vi "widget.vi"() -> ()   [LabVIEW 2018]
uses:
  <vilib>/Instr/_visa.llb/VISA Configure Serial Port (Instr).vi
  PCI8552B_32.dll
panel:
  out "待读取数据长度":i32
  out "步进电机步进次数":dbl
  out "频率步进次数":dbl
  in  "步进电机确定":bool
  in  "频率确定":bool
  in  "开关确定":bool
  in  "开始":bool
  in  "停止":bool
  in  "扫描模式":u16(ring)=2 items=["多频多角度模式", "校正模式", "单点模式", "单列模式", "单频多角度模式"]
  out "ch1":dbl[](graph)
  out "ch0":dbl[](graph)
  out "采集卡状态":bool
  out "开关控制器状态":bool
  out "步进电机控制器状态":bool
  in  "物体距离":dbl=150.0
  in  "频率间隔":dbl=0.1
  in  "步进间隔":dbl=5.0
  in  "移动坐标":dbl
  in  "改变频率":dbl
  in  "切换开关":dbl
  out "当前位置":dbl format="%#_4f"
  out "当前开关":dbl=1.0
  out "当前频率":dbl=24.0
  in  "开关控制器":refnum<visa-resource-name>
  in  "步进电机控制器":refnum<visa-resource-name>
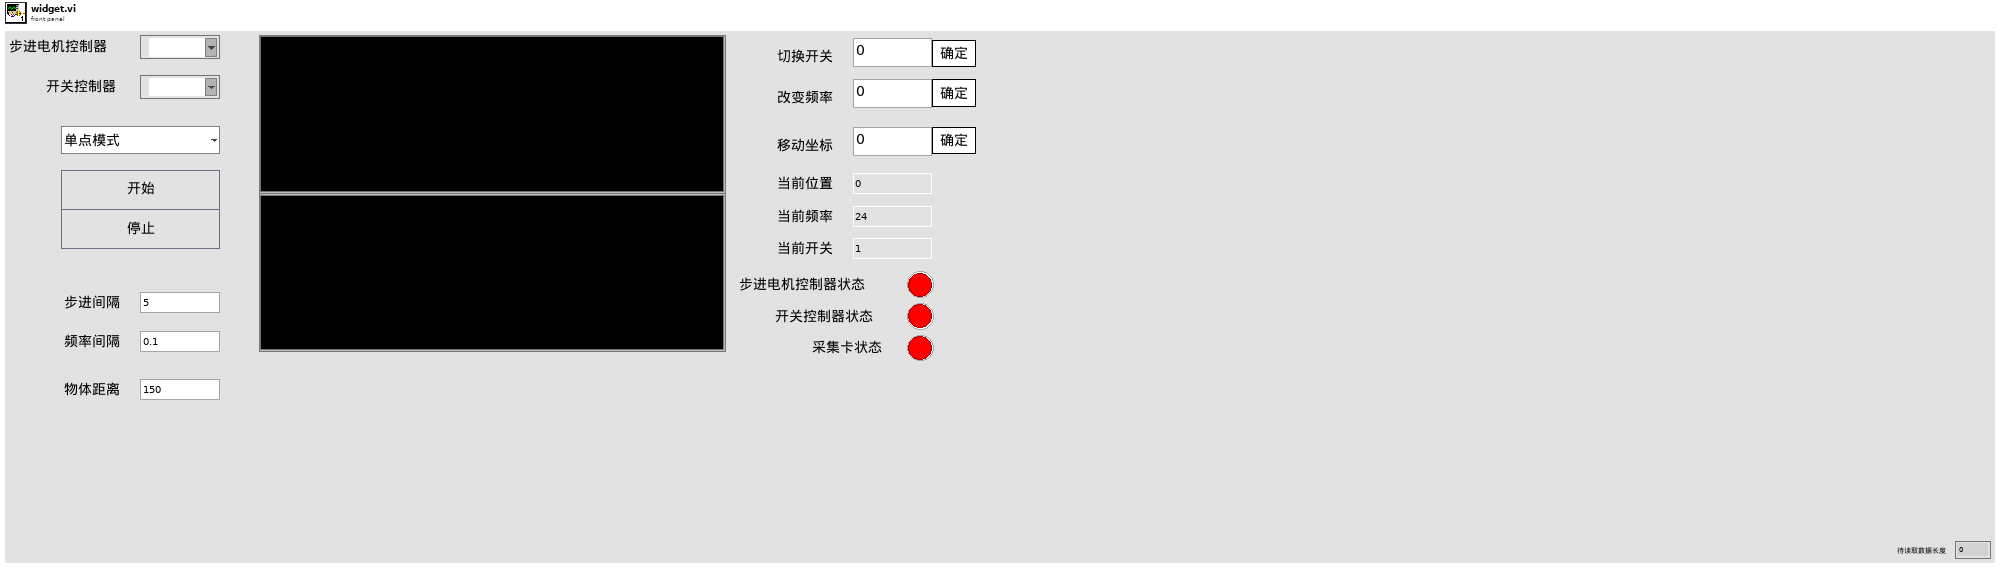
[diagram p1: front panel]
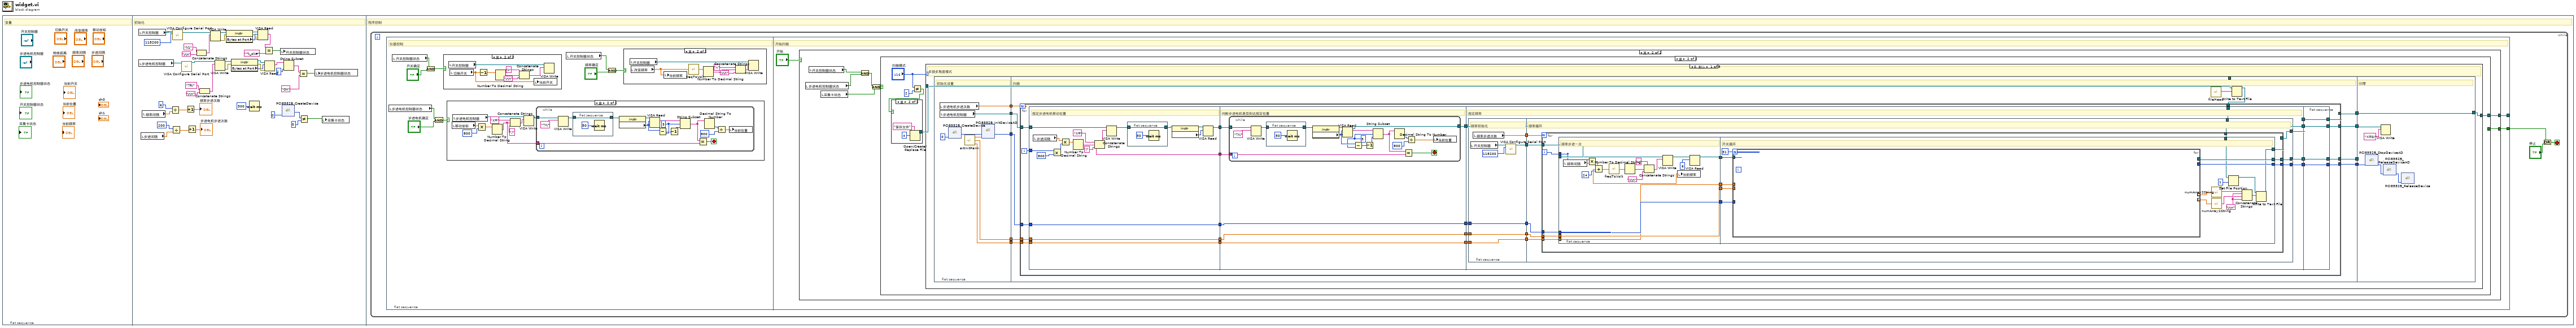
[diagram p0: block diagram]
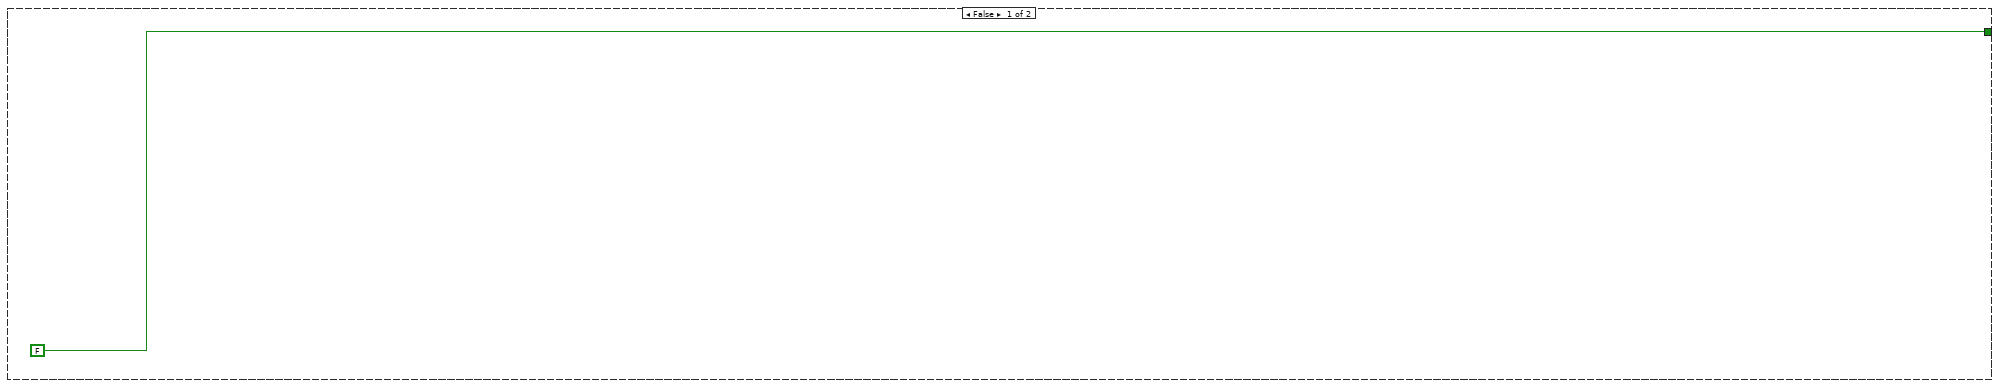
[diagram p5: hidden frame]
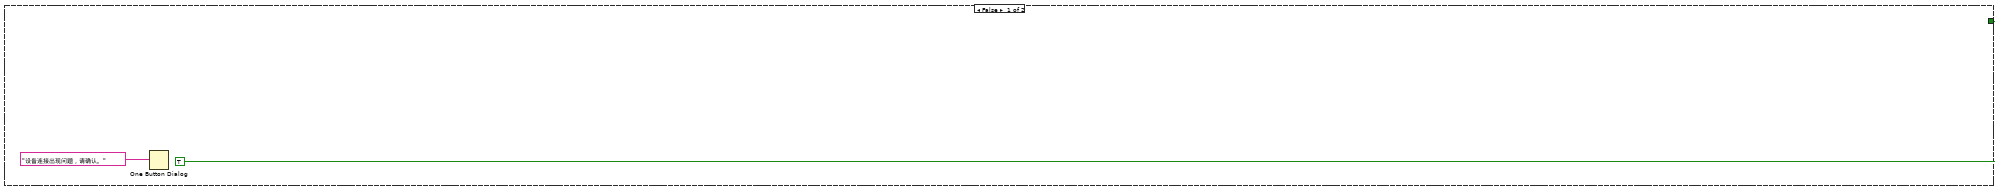
[diagram p6: hidden frame]
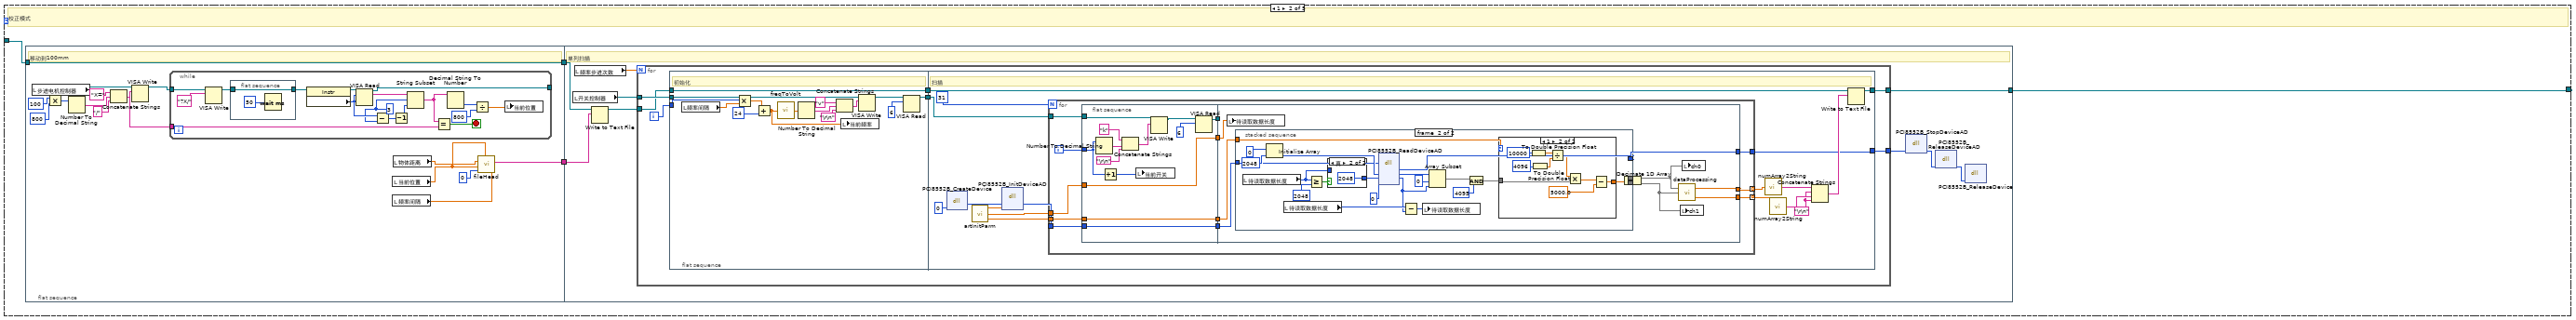
[diagram p8: hidden frame]
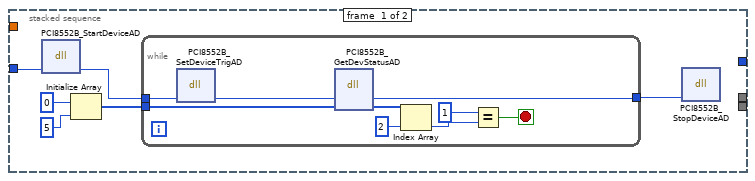
[diagram p9: hidden frame]
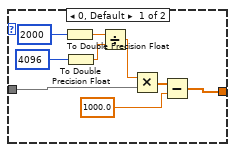
[diagram p10: hidden frame]
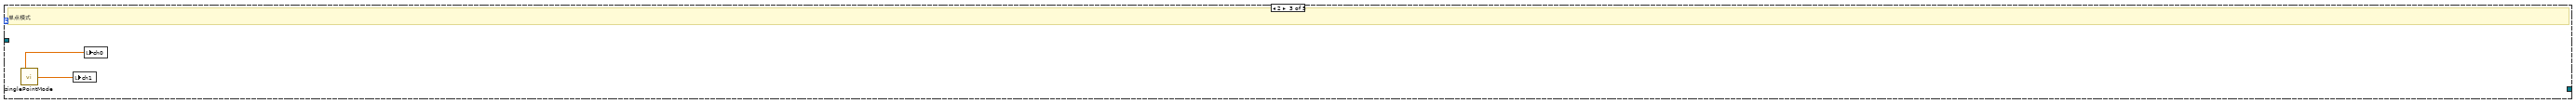
[diagram p12: hidden frame]
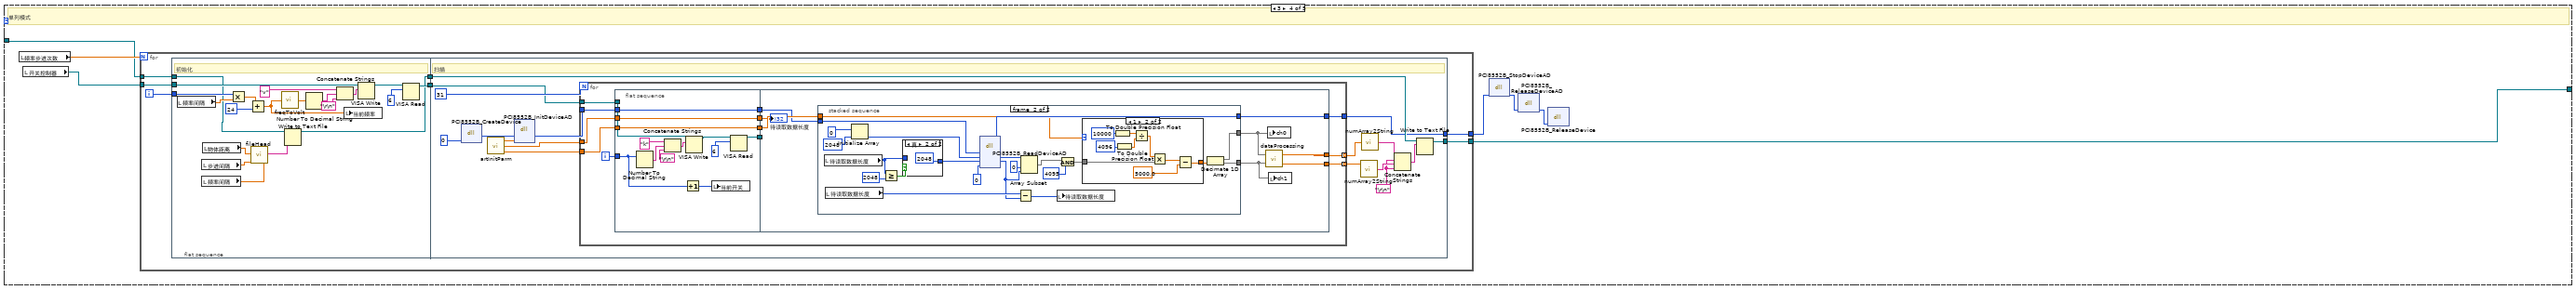
[diagram p13: hidden frame]
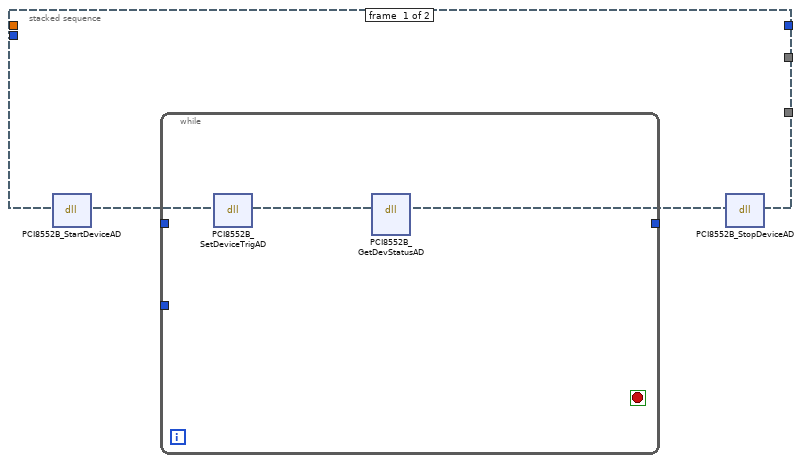
[diagram p14: hidden frame]
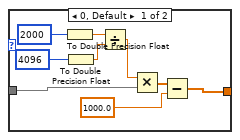
[diagram p15: hidden frame]
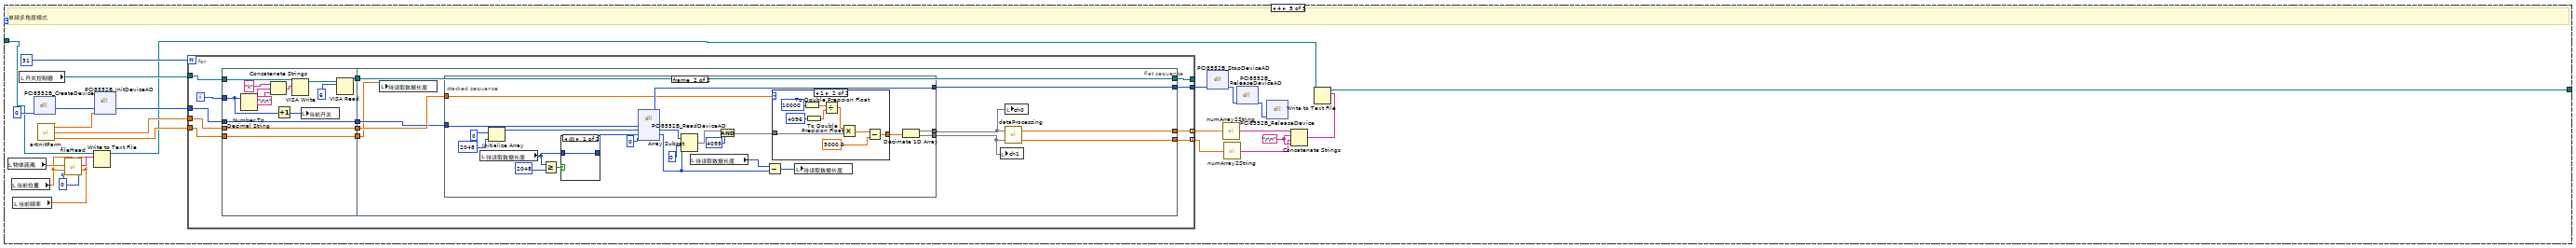
[diagram p17: hidden frame]
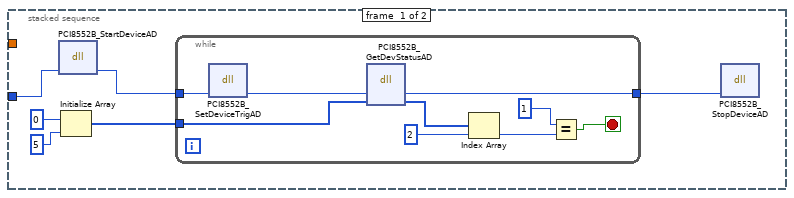
[diagram p18: hidden frame]
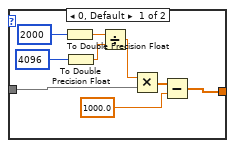
[diagram p19: hidden frame]
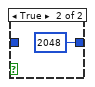
[diagram p20: hidden frame]
diagram:
  n1 = flat-sequence {
    frame #0 {
      # "变量"
    }
    frame #1 {
      # "初始化"
      n2 = local read "开关控制器"() -> (w23:refnum<visa-resource-name>)
      n3 = local read "步进电机控制器"() -> (w20:refnum<visa-resource-name>)
      n4 = local read "步进间隔"() -> (w3:dbl)
      n5 = local read "频率间隔"() -> (w7:dbl)
      n6 = Divide(x=6, y=w7) -> (x/y=w6:dbl)
      n7 = Divide(x=200, y=w3) -> (x/y=w2:dbl)
      n8 = call-poly "VISA Configure Serial Port"("VISA resource name"=w23, "baud rate (9600)"=115200) -> ("VISA resource name out"=w22:refnum<visa-resource-name>)  [unwired: 12 in, 1 out]
      n9 = call-poly "VISA Configure Serial Port"("VISA resource name"=w20) -> ("VISA resource name out"=w19:refnum<visa-resource-name>)  [unwired: 13 in, 1 out]
      n10 = Increment(x=w6) -> (x+1=→"频率步进次数":dbl)
      n11 = Increment(x=w2) -> (x+1=→"步进电机步进次数":dbl)
      n12 = Concatenate Strings("k1", "\r\n") -> (w40:string)
      n13 = Concatenate Strings("?R/", "\r\n") -> (w14:string)
      n14 = VISA Write(VISA resource name=w22, write buffer=w40) -> (VISA resource name out=w39:refnum<visa-resource-name>, error out=w29:errorcluster)  [unwired: 1 in, 1 out]
      n15 = VISA Write(VISA resource name=w19, write buffer=w14) -> (VISA resource name out=w34:refnum<visa-resource-name>, error out=w33:errorcluster)  [unwired: 1 in, 1 out]
      n16 = property class="Instr"(reference=w39, error in=w29) -> (reference out=w38:refnum<visa-resource-name>, error out=w28:errorcluster, "Bytes at Port"=w37:u32)
      n17 = property class="Instr"(reference=w34, error in=w33) -> (reference out=w30:refnum<visa-resource-name>, error out=w32:errorcluster, "Bytes at Port"=w31:u32)
      n18 = Wait (ms)(milliseconds to wait=300) -> ()  [unwired: 1 out]
      n19 = VISA Read(VISA resource name=w38, byte count=w37, error in (no error)=w28) -> (read buffer=w18:string)  [unwired: 3 out]
      n20 = Equal?(x=w18, y="*k_ok#") -> (x = y?=w35:bool)
      n21 = VISA Read(VISA resource name=w30, byte count=w31, error in (no error)=w32) -> (read buffer=w27:string)  [unwired: 3 out]
      n22 = local write "开关控制器状态"(w35) -> ()
      n23 = dll-call lib="C:/Users/BlueMess/Desktop/Work2020/MMW Controller/mmw_controller/PCI8552B_32.dll" fn="PCI8552B_CreateDevice" label="CreateDevice"("DeviceLgcID"=0) -> ("返回类型"=w11:i32)  [unwired: 4 in, 2 out]
      n24 = String Subset(string=w27, length (rest)=2) -> (substring=w17:string)  [unwired: 1 in]
      n25 = Equal?(x=w17, y="OK") -> (x = y?=w24:bool)
      n26 = Not Equal?(x=w11, y=0 ("DeviceLgcID")) -> (x != y?=w12:bool)
      n27 = local write "步进电机控制器状态"(w24) -> ()
      n28 = local write "采集卡状态"(w12) -> ()
    }
    frame #2 {
      # "程序控制"
      n29 = while {
        stop <- w43 stop-if-true
        n30 = flat-sequence {
          tunnel: [w98] -> w45
          tunnel: [w96] -> _
          frame #0 {
            # "仪器控制"
            n31 = local read "步进电机控制器状态"() -> (w48:bool)
            n32 = local read "开关控制器状态"() -> (w54:bool)
            n33 = And(x=w54, y="开关确定") -> (x .and. y?=w52:bool)
            n34 = And(x=w48, y="步进电机确定") -> (x .and. y?=w46:bool)
            n35 = case shown="真" w52 {
              frame False {
              }
              frame True {
                n36 = local read "开关控制器"() -> (w93:refnum<visa-resource-name>)
                n37 = local read "切换开关"() -> (w89:dbl)
                n38 = Decrement(x=w89) -> (x-1=w90:dbl)
                n39 = Number To Decimal String(number=w90) -> (decimal integer string=w91:string)  [unwired: 1 in]
                n40 = Concatenate Strings("k", w91, "\r\n") -> (w94:string)
                n41 = local write "当前开关"(w89) -> ()
                n42 = VISA Write(VISA resource name=w93, write buffer=w94) -> ()  [unwired: 1 in, 3 out]
              }
            }
            n43 = case shown="真" w46 {
              frame False {
              }
              frame True {
                n44 = local read "移动坐标"() -> (w61:dbl)
                n45 = local read "步进电机控制器"() -> (w63:refnum<visa-resource-name>)
                n46 = Multiply(x=w61, y=800) -> (x*y=w59:dbl)
                n47 = Number To Decimal String(number=w59) -> (decimal integer string=w55:string)  [unwired: 1 in]
                n48 = Concatenate Strings("X=", w55, "/") -> (w57:string)
                n49 = VISA Write(VISA resource name=w63, write buffer=w57) -> (VISA resource name out=w56:refnum<visa-resource-name>)  [unwired: 1 in, 2 out]
                n50 = while {
                  tunnel: w56 -> [w79]
                  tunnel: w55 -> [w69]
                  stop <- w68 stop-if-true
                  w72 = 3
                  n51 = VISA Write(VISA resource name=w79, write buffer="?X/") -> (VISA resource name out=w77:refnum<visa-resource-name>)  [unwired: 1 in, 2 out]
                  n52 = flat-sequence {
                    tunnel: w77 -> [w80]
                    tunnel: [w80] -> w76
                    frame #0 {
                      n53 = Wait (ms)(milliseconds to wait=50) -> ()  [unwired: 1 out]
                    }
                  }
                  n54 = property class="Instr"(reference=w76) -> (reference out=w75:refnum<visa-resource-name>, "Serial Settings:Number of Bytes at Serial Port"=w73:u32)  [unwired: 1 in, 1 out]
                  n55 = VISA Read(VISA resource name=w75, byte count=w73) -> (read buffer=w74:string)  [unwired: 1 in, 3 out]
                  n56 = Subtract(x=w73, y=w72) -> (x-y=w71:u32)
                  n57 = Decrement(x=w71) -> (x-1=w70:u32)
                  n58 = String Subset(string=w74, offset (0)=w72, length (rest)=w70) -> (substring=w67:string)
                  n59 = Equal?(x=w67, y=w69) -> (x = y?=w68:bool)
                  n60 = Decimal String To Number(string=w67) -> (number=w66:i32)  [unwired: 2 in, 1 out]
                  n61 = Divide(x=w66, y=800) -> (x/y=w64:dbl)
                  n62 = local write "当前位置"(w64) -> ()
                }
              }
            }
            n63 = local read "开关控制器状态"() -> (w51:bool)
            n64 = And(x=w51, y="频率确定") -> (x .and. y?=w49:bool)
            n65 = case shown="真" w49 {
              frame False {
              }
              frame True {
                n66 = local read "开关控制器"() -> (w85:refnum<visa-resource-name>)
                n67 = local read "改变频率"() -> (w82:dbl)
                n68 = local write "当前频率"(w82) -> ()
                n69 = call "freqToVolt.vi"("频率"=w82) -> ("电压"=w84:dbl)
                n70 = Number To Decimal String(number=w84) -> (decimal integer string=w86:string)  [unwired: 1 in]
                n71 = Concatenate Strings("v", w86, "\r\n") -> (w83:string)
                n72 = VISA Write(VISA resource name=w85, write buffer=w83) -> ()  [unwired: 1 in, 3 out]
              }
            }
          }
          frame #1 {
            # "开始扫描"
            n73 = case shown="真" "开始" {
              tunnel: [FALSE w106] -> w98
              tunnel: [_ w100] -> w96
              frame False {
              }
              frame True {
                n74 = local read "步进电机控制器状态"() -> (w104:bool)
                n75 = local read "开关控制器状态"() -> (w105:bool)
                n76 = local read "采集卡状态"() -> (w102:bool)
                n77 = And(x=w105, y=w104) -> (x .and. y?=w103:bool)
                n78 = And(x=w103, y=w102) -> (x .and. y?=w101:bool)
                n79 = case shown="真" w101 {
                  tunnel: [TRUE _] -> w106
                  tunnel: [_ w112] -> w100
                  frame False {
                    n80 = One Button Dialog(message="设备连接出现问题，请确认。") -> ()  [unwired: 1 in, 1 out]
                  }
                  frame True {
                    n81 = Not Equal?(x="扫描模式", y=2) -> (x != y?=w109:bool)
                    n82 = case shown="真" w109 {
                      tunnel: [_ w115] -> w113
                      frame False {
                      }
                      frame True {
                        n83 = Open/Create/Replace File(prompt="保存文件", operation (0:open)=4) -> (refnum out=w115:refnum<file>)  [unwired: 4 in, 2 out]
                      }
                    }
                    n84 = case shown="0, 默认" "扫描模式" {
                      tunnel: w113 -> [w117 w396 _ w576 w719]
                      tunnel: [w118 w395 _ w572 w723] -> w112
                      frame 0, Default {
                        # "多频多角度模式"
                        n85 = flat-sequence {
                          tunnel: [w128] -> w127
                          tunnel: [w129] -> w126
                          tunnel: [w132] -> w125
                          tunnel: [w131] -> w124
                          tunnel: [w130] -> w123
                          tunnel: w127 -> [w147]
                          tunnel: w126 -> [w146]
                          tunnel: [w145] -> w122
                          tunnel: [w144] -> w121
                          tunnel: w125 -> [w143]
                          tunnel: w124 -> [w142]
                          tunnel: w123 -> [w141]
                          tunnel: [w140] -> w120
                          tunnel: [w139] -> w119
                          tunnel: w117 -> [w138]
                          tunnel: w122 -> [w392]
                          tunnel: w121 -> [_]
                          tunnel: w120 -> [w389]
                          tunnel: w119 -> [w388]
                          tunnel: [w388] -> w118
                          frame #0 {
                            # "初始化设置"
                            n86 = local read "步进电机步进次数"() -> (w128:dbl)
                            n87 = local read "步进电机控制器"() -> (w129:refnum<visa-resource-name>)
                            n88 = dll-call lib="C:/Users/BlueMess/Desktop/Work2020/MMW Controller/mmw_controller/PCI8552B_32.dll" fn="PCI8552B_CreateDevice" label="CreateDevice"("DeviceLgcID"=0) -> ("返回类型"=w134:i32)  [unwired: 4 in, 2 out]
                            n89 = call "artInitParm.vi"() -> ("待读取长度"=w130:dbl, "量程选择"=w131:dbl, "初始化参数"=w135:dbl[])
                            n90 = dll-call lib="C:/Users/BlueMess/Desktop/Work2020/MMW Controller/mmw_controller/PCI8552B_32.DLL" fn="PCI8552B_InitDeviceAD" label="InitDeviceAD"("hDevice"=w134, "pADPara"=w135) -> ("hDevice"=w132:i32)  [unwired: 5 in, 2 out]
                          }
                          frame #1 {
                            # "扫描"
                            n91 = call "fileHead.vi"() -> ("输出"=w136:string)  [unwired: 9 in]
                            n92 = Write to Text File(file (use dialog)=w138, text=w136) -> (refnum out=w137:refnum<file>)  [unwired: 2 in, 2 out]
                            n93 = for {
                              N: w147 -> [_]
                              tunnel: w146 -> [w169]
                              tunnel: [w164] -> w145
                              tunnel: [w162] -> w144
                              tunnel: w143 -> [w160]
                              tunnel: w142 -> [w158]
                              tunnel: w141 -> [w156]
                              tunnel: [w151] -> w140
                              tunnel: [w149] -> w139
                              tunnel: w137 -> [w148]
                              i -> [w170]
                              n94 = flat-sequence "平铺式顺序结构" {
                                tunnel: w170 -> [w171]
                                tunnel: w169 -> [w184]
                                tunnel: [w177] -> w168
                                tunnel: [w175] -> w167
                                tunnel: [w174] -> w161
                                tunnel: w160 -> [w174]
                                tunnel: [w173] -> w159
                                tunnel: w158 -> [w173]
                                tunnel: [w172] -> w157
                                tunnel: w156 -> [w172]
                                tunnel: w168 -> [w196]
                                tunnel: w167 -> [w195]
                                tunnel: [w194] -> w165
                                tunnel: w161 -> [w193]
                                tunnel: w159 -> [w192]
                                tunnel: w157 -> [w191]
                                tunnel: [w193] -> w155
                                tunnel: [w192] -> w154
                                tunnel: [w191] -> w153
                                tunnel: [w228] -> w166
                                tunnel: w165 -> [w228]
                                tunnel: [w225] -> w163
                                tunnel: w155 -> [w223]
                                tunnel: w154 -> [w221]
                                tunnel: w153 -> [w219]
                                tunnel: [w218] -> w152
                                tunnel: [w217] -> w150
                                tunnel: w148 -> [w216]
                                tunnel: w166 -> [w387]
                                tunnel: [w387] -> w164
                                tunnel: w163 -> [w386]
                                tunnel: [w386] -> w162
                                tunnel: w152 -> [w385]
                                tunnel: [w385] -> w151
                                tunnel: [w384] -> w149
                                tunnel: w150 -> [w384]
                                frame #0 {
                                # "指定步进电机移动位置"
                                n95 = local read "步进间隔"() -> (w187:dbl)
                                n96 = Multiply(x=w171, y=800) -> (x*y=w186:i32)
                                n97 = Multiply(x=w187, y=w186) -> (x*y=w185:dbl)
                                n98 = Number To Decimal String(number=w185) -> (decimal integer string=w175:string)  [unwired: 1 in]
                                n99 = Concatenate Strings("X=", w175, "/") -> (w176:string)
                                n100 = VISA Write(VISA resource name=w184, write buffer=w176) -> (VISA resource name out=w181:refnum<visa-resource-name>)  [unwired: 1 in, 2 out]
                                n101 = flat-sequence {
                                tunnel: w181 -> [w189]
                                tunnel: [w189] -> w180
                                frame #0 {
                                n102 = Wait (ms)(milliseconds to wait=50) -> ()  [unwired: 1 out]
                                }
                                }
                                n103 = property class="Instr"(reference=w180) -> (reference out=w179:refnum<visa-resource-name>, "Serial Settings:Number of Bytes at Serial Port"=w178:u32)  [unwired: 1 in, 1 out]
                                n104 = VISA Read(VISA resource name=w179, byte count=w178) -> (VISA resource name out=w177:refnum<visa-resource-name>)  [unwired: 1 in, 3 out]
                                }
                                frame #1 {
                                # "判断步进电机是否到达指定位置"
                                n105 = while {
                                tunnel: w196 -> [w213]
                                tunnel: w195 -> [w203]
                                tunnel: [w201] -> w194
                                stop <- w202 stop-if-true
                                w206 = 3
                                n106 = VISA Write(VISA resource name=w213, write buffer="?X/") -> (VISA resource name out=w211:refnum<visa-resource-name>)  [unwired: 1 in, 2 out]
                                n107 = flat-sequence {
                                tunnel: w211 -> [w214]
                                tunnel: [w214] -> w210
                                frame #0 {
                                n108 = Wait (ms)(milliseconds to wait=50) -> ()  [unwired: 1 out]
                                }
                                }
                                n109 = property class="Instr"(reference=w210) -> (reference out=w209:refnum<visa-resource-name>, "Serial Settings:Number of Bytes at Serial Port"=w207:u32)  [unwired: 1 in, 1 out]
                                n110 = VISA Read(VISA resource name=w209, byte count=w207) -> (VISA resource name out=w201:refnum<visa-resource-name>, read buffer=w208:string)  [unwired: 1 in, 2 out]
                                n111 = Subtract(x=w207, y=w206) -> (x-y=w205:u32)
                                n112 = Decrement(x=w205) -> (x-1=w204:u32)
                                n113 = String Subset(string=w208, offset (0)=w206, length (rest)=w204) -> (substring=w200:string)
                                n114 = Decimal String To Number(string=w200) -> (number=w199:i32)  [unwired: 2 in, 1 out]
                                n115 = Equal?(x=w200, y=w203) -> (x = y?=w202:bool)
                                n116 = Divide(x=w199, y=800) -> (x/y=w197:dbl)
                                n117 = local write "当前位置"(w197) -> ()
                                }
                                }
                                frame #2 {
                                # "指定频率"
                                n118 = flat-sequence {
                                tunnel: [w233] -> w227
                                tunnel: [w232] -> w226
                                tunnel: [w231] -> w224
                                tunnel: w223 -> [w231]
                                tunnel: [w230] -> w222
                                tunnel: w221 -> [w230]
                                tunnel: [w229] -> w220
                                tunnel: w219 -> [w229]
                                tunnel: w227 -> [w244]
                                tunnel: w226 -> [w243]
                                tunnel: [w242] -> w225
                                tunnel: w224 -> [w241]
                                tunnel: w222 -> [w240]
                                tunnel: w220 -> [w239]
                                tunnel: [w238] -> w218
                                tunnel: [w237] -> w217
                                tunnel: w216 -> [w236]
                                frame #0 {
                                # "频率初始化"
                                n119 = local read "开关控制器"() -> (w234:refnum<visa-resource-name>)
                                n120 = local read "频率步进次数"() -> (w233:dbl)
                                n121 = call-poly "VISA Configure Serial Port"("VISA resource name"=w234, "baud rate (9600)"=115200) -> ("VISA resource name out"=w232:refnum<visa-resource-name>)  [unwired: 12 in, 1 out]
                                }
                                frame #1 {
                                # "频率循环"
                                n122 = for {
                                N: w244 -> [_]
                                tunnel: w243 -> [w257]
                                tunnel: [w255] -> w242
                                tunnel: w241 -> [w253]
                                tunnel: w240 -> [w251]
                                tunnel: w239 -> [w249]
                                tunnel: [w248] -> w238
                                tunnel: [w247] -> w237
                                tunnel: w236 -> [w245]
                                i -> [w246]
                                n123 = flat-sequence {
                                tunnel: [w258] -> _
                                tunnel: w257 -> [w271]
                                tunnel: [w267] -> w256
                                tunnel: [w262] -> w254
                                tunnel: w253 -> [w262]
                                tunnel: [w261] -> w252
                                tunnel: w251 -> [w261]
                                tunnel: [w260] -> w250
                                tunnel: w249 -> [w260]
                                tunnel: w246 -> [w258]
                                tunnel: w256 -> [w290]
                                tunnel: [w289] -> w255
                                tunnel: w254 -> [w288]
                                tunnel: w252 -> [w287]
                                tunnel: w250 -> [w286]
                                tunnel: [w283] -> w248
                                tunnel: [w282] -> w247
                                tunnel: w245 -> [w277]
                                frame #0 {
                                # "频率步进一次"
                                n124 = local read "频率间隔"() -> (w274:dbl)
                                n125 = Multiply(x=w258, y=w274) -> (x*y=w273:dbl)
                                n126 = Add(x=w273, y=24) -> (x+y=w259:dbl)
                                n127 = call "freqToVolt.vi"("频率"=w259) -> ("电压"=w265:dbl)
                                n128 = Number To Decimal String(number=w265) -> (decimal integer string=w269:string)  [unwired: 1 in]
                                n129 = Concatenate Strings("v", w269, "\r\n") -> (w266:string)
                                n130 = VISA Write(VISA resource name=w271, write buffer=w266) -> (VISA resource name out=w264:refnum<visa-resource-name>)  [unwired: 1 in, 2 out]
                                n131 = local write "当前频率"(w259) -> ()
                                n132 = VISA Read(VISA resource name=w264, byte count=6) -> (VISA resource name out=w267:refnum<visa-resource-name>)  [unwired: 1 in, 3 out]
                                }
                                frame #1 {
                                w281 = "\r\n"
                                # "开关循环"
                                n133 = for {
                                N: 31 -> [_]
                                tunnel: w290 -> [w304]
                                tunnel: [w303] -> w289
                                tunnel: w288 -> [w299]
                                tunnel: w287 -> [w297]
                                tunnel: w286 -> [w295]
                                tunnel: [w294] -> w283
                                tunnel: [w293] -> w278 mode=indexing
                                tunnel: [w292] -> w279 mode=indexing
                                i -> [w302]
                                n134 = flat-sequence {
                                tunnel: w304 -> [w317]
                                tunnel: w302 -> [w305]
                                tunnel: [w312] -> w301
                                tunnel: [w309] -> w300
                                tunnel: w299 -> [w309]
                                tunnel: [w308] -> w298
                                tunnel: w297 -> [w308]
                                tunnel: [w307] -> w296
                                tunnel: w295 -> [w307]
                                tunnel: [w326] -> w303
                                tunnel: w301 -> [w326]
                                tunnel: w300 -> [w324]
                                tunnel: w298 -> [w325]
                                tunnel: w296 -> [w320]
                                tunnel: [w323] -> w294
                                tunnel: [w322] -> w293
                                tunnel: [w321] -> w292
                                frame #0 {
                                n135 = Number To Decimal String(number=w305) -> (decimal integer string=w316:string)  [unwired: 1 in]
                                n136 = Increment(x=w305) -> (x+1=w306:i32)
                                n137 = Concatenate Strings("k", w316, "\r\n") -> (w313:string)
                                n138 = VISA Write(VISA resource name=w317, write buffer=w313) -> (VISA resource name out=w311:refnum<visa-resource-name>)  [unwired: 1 in, 2 out]
                                n139 = local write "当前开关"(w306) -> ()
                                n140 = VISA Read(VISA resource name=w311, byte count=6) -> (VISA resource name out=w312:refnum<visa-resource-name>)  [unwired: 1 in, 3 out]
                                }
                                frame #1 {
                                n141 = local write "待读取数据长度"(w320) -> ()
                                n142 = stacked-sequence {
                                tunnel: w324 -> [w328 w359]
                                tunnel: [_ w363] -> w323
                                tunnel: w325 -> [_ w358]
                                tunnel: [_ w357] -> w319
                                tunnel: [_ w356] -> w318
                                frame #0 {
                                n143 = dll-call lib="C:/Users/BlueMess/Desktop/Work2020/MMW Controller/mmw_controller/PCI8552B_32.DLL" fn="PCI8552B_StartDeviceAD" label="StartDeviceAD"("hDevice"=w328) -> ("hDevice"=w327:i32)  [unwired: 4 in, 2 out]
                                n144 = Initialize Array(0, 5) -> (w332:i32[])
                                n145 = while {
                                tunnel: w327 -> [w336]
                                tunnel: w332 -> [w341]
                                tunnel: [w334] -> w329
                                stop <- w333 stop-if-true
                                n146 = dll-call lib="C:/Users/BlueMess/Desktop/Work2020/MMW Controller/mmw_controller/PCI8552B_32.DLL" fn="PCI8552B_SetDeviceTrigAD" label="SetDeviceTrigAD"("hDevice"=w336) -> ("hDevice"=w335:i32)  [unwired: 4 in, 2 out]
                                n147 = dll-call lib="C:/Users/BlueMess/Desktop/Work2020/MMW Controller/mmw_controller/PCI8552B_32.DLL" fn="PCI8552B_GetDevStatusAD" label="GetDevStatusAD"("hDevice"=w335, "ADStatus"=w341) -> ("hDevice"=w334:i32, "ADStatus"=w337:i32[])  [unwired: 4 in, 2 out]
                                n148 = Index Array(array=w337, index=2) -> (element=w339:i32)
                                n149 = Equal?(x=1, y=w339) -> (x = y?=w333:bool)
                                }
                                n150 = dll-call lib="C:/Users/BlueMess/Desktop/Work2020/MMW Controller/mmw_controller/PCI8552B_32.DLL" fn="PCI8552B_StopDeviceAD" label="StopDeviceAD"("hDevice"=w329) -> ()  [unwired: 5 in, 2 out]
                                }
                                frame #1 {
                                n151 = local read "待读取数据长度"() -> (w353:i32)
                                n152 = Initialize Array(u16 0 ("y"), 2048 ("y")) -> (w360:u16[])
                                n153 = Greater Or Equal?(x=w353, y=2048 ("millisecond multiple")) -> (x >= y?=w354:bool)
                                n154 = case shown="真" w354 {
                                tunnel: [w382 2048 ("millisecond multiple")] -> w351
                                tunnel: w353 -> [w382 _]
                                frame False {
                                }
                                frame True {
                                }
                                }
                                n155 = local read "待读取数据长度"() -> (w342:i32)
                                n156 = dll-call lib="C:/Users/BlueMess/Desktop/Work2020/MMW Controller/mmw_controller/PCI8552B_32.DLL" fn="PCI8552B_ReadDeviceAD" label="ReadDeviceAD"("hDevice"=w359, "pADBuffer"=w360, "nReadSizeWords"=w351, "nRetSizeWords"=0) -> ("hDevice"=w363:i32, "pADBuffer"=w346:u16[], "nReadSizeWords"=w343:u32)  [unwired: 5 in, 2 out]
                                n157 = Subtract(x=w342, y=w343) -> (x-y=w352:u32)
                                n158 = Array Subset(array=w346, index=0 ("索引"), length=w343) -> (w345:u16[])
                                n159 = local write "待读取数据长度"(w352) -> ()
                                n160 = And(x=w345, y=u16 4095) -> (x .and. y?=w349:u16[])
                                n161 = case shown="0, 默认" w358 {
                                tunnel: w349 -> [w371 w376]
                                tunnel: [w364 w375] -> w348
                                frame 0, Default {
                                n162 = To Double Precision Float(number=2000 ("x")) -> (double precision float=w367:dbl)
                                n163 = To Double Precision Float(number=4096) -> (double precision float=w366:dbl)
                                n164 = Divide(x=w367, y=w366) -> (x/y=w372:dbl)
                                n165 = Multiply(x=w372, y=w371) -> (x*y=w370:dbl[])
                                n166 = Subtract(x=w370, y=1000.0) -> (x-y=w364:dbl[])
                                }
                                frame 1 {
                                n167 = To Double Precision Float(number=10000 ("x")) -> (double precision float=w374:dbl)
                                n168 = To Double Precision Float(number=4096) -> (double precision float=w378:dbl)
                                n169 = Divide(x=w374, y=w378) -> (x/y=w381:dbl)
                                n170 = Multiply(x=w381, y=w376) -> (x*y=w380:dbl[])
                                n171 = Subtract(x=w380, y=5000.0) -> (x-y=w375:dbl[])
                                }
                                }
                                n172 = Decimate 1D Array(w348) -> (w357:dbl[], w356:dbl[])
                                }
                                }
                                n173 = local write "ch0"(w319) -> ()
                                n174 = local write "ch1"(w318) -> ()
                                n175 = call "dataProcessing.vi"("中频信号"=w318, "参考信号"=w319) -> ("mean_Q"=w321:dbl, "mean_I"=w322:dbl)
                                }
                                }
                                }
                                n176 = call "numArray2String.vi"("输入数组"=w278) -> ("输出字符串"=w275:string)
                                n177 = call "numArray2String.vi"("输入数组"=w279) -> ("输出字符串"=w276:string)
                                n178 = Set File Position(refnum=w277, from (0:start)=1) -> (refnum out=w285:refnum<file>)  [unwired: 2 in, 1 out]
                                n179 = Concatenate Strings(w275, w281, w276, w281) -> (w280:string)
                                n180 = Write to Text File(file (use dialog)=w285, text=w280) -> (refnum out=w282:refnum<file>)  [unwired: 2 in, 2 out]
                                }
                                }
                                }
                                }
                                }
                                }
                                frame #3 {
                                }
                              }
                            }
                          }
                          frame #2 {
                            # "归零"
                            n181 = dll-call lib="C:/Users/BlueMess/Desktop/Work2020/MMW Controller/mmw_controller/PCI8552B_32.DLL" fn="PCI8552B_StopDeviceAD" label="StopDeviceAD"("hDevice"=w389) -> ("hDevice"=w391:i32)  [unwired: 4 in, 2 out]
                            n182 = VISA Write(VISA resource name=w392, write buffer="X=0/") -> ()  [unwired: 1 in, 3 out]
                            n183 = dll-call lib="C:/Users/BlueMess/Desktop/Work2020/MMW Controller/mmw_controller/PCI8552B_32.DLL" fn="PCI8552B_ReleaseDeviceAD" label="ReleaseDeviceAD"("hDevice"=w391) -> ("hDevice"=w390:i32)  [unwired: 4 in, 2 out]
                            n184 = dll-call lib="C:/Users/BlueMess/Desktop/Work2020/MMW Controller/mmw_controller/PCI8552B_32.DLL" fn="PCI8552B_ReleaseDevice" label="ReleaseDevice"("hDevice"=w390) -> ()  [unwired: 5 in, 2 out]
                          }
                        }
                      }
                      frame 1 {
                        # "校正模式"
                        n185 = flat-sequence {
                          tunnel: [w403] -> w397
                          tunnel: w396 -> [w403]
                          tunnel: [w402] -> w394
                          tunnel: w397 -> [w434]
                          tunnel: [w435] -> w395
                          tunnel: w394 -> [w432]
                          frame #0 {
                            # "移动到100mm"
                            n186 = local read "步进电机控制器"() -> (w405:refnum<visa-resource-name>)
                            n187 = Multiply(x=100, y=800) -> (x*y=w408:i32)
                            n188 = Number To Decimal String(number=w408) -> (decimal integer string=w412:string)  [unwired: 1 in]
                            n189 = Concatenate Strings("X=", w412, "/") -> (w410:string)
                            n190 = VISA Write(VISA resource name=w405, write buffer=w410) -> (VISA resource name out=w411:refnum<visa-resource-name>)  [unwired: 1 in, 2 out]
                            n191 = while {
                              tunnel: w411 -> [w429]
                              tunnel: w412 -> [w419]
                              tunnel: [w417] -> _
                              stop <- w418 stop-if-true
                              w422 = 3
                              n192 = VISA Write(VISA resource name=w429, write buffer="?X/") -> (VISA resource name out=w427:refnum<visa-resource-name>)  [unwired: 1 in, 2 out]
                              n193 = flat-sequence {
                                tunnel: w427 -> [w430]
                                tunnel: [w430] -> w426
                                frame #0 {
                                n194 = Wait (ms)(milliseconds to wait=50) -> ()  [unwired: 1 out]
                                }
                              }
                              n195 = property class="Instr"(reference=w426) -> (reference out=w425:refnum<visa-resource-name>, "Serial Settings:Number of Bytes at Serial Port"=w423:u32)  [unwired: 1 in, 1 out]
                              n196 = VISA Read(VISA resource name=w425, byte count=w423) -> (VISA resource name out=w417:refnum<visa-resource-name>, read buffer=w424:string)  [unwired: 1 in, 2 out]
                              n197 = Subtract(x=w423, y=w422) -> (x-y=w421:u32)
                              n198 = Decrement(x=w421) -> (x-1=w420:u32)
                              n199 = String Subset(string=w424, offset (0)=w422, length (rest)=w420) -> (substring=w416:string)
                              n200 = Equal?(x=w416, y=w419) -> (x = y?=w418:bool)
                              n201 = Decimal String To Number(string=w416) -> (number=w415:i32)  [unwired: 2 in, 1 out]
                              n202 = Divide(x=w415, y=800) -> (x/y=w413:dbl)
                              n203 = local write "当前位置"(w413) -> ()
                            }
                            n204 = local read "当前位置"() -> (w399:dbl)
                            n205 = local read "频率间隔"() -> (w398:dbl)
                            n206 = local read "物体距离"() -> (w401:dbl)
                            n207 = call "fileHead.vi"("df"=w398, "x_max"=w399, "dx"=0, "x_min"=w399, "distance"=w401) -> ("输出"=w402:string)  [unwired: 4 in]
                          }
                          frame #1 {
                            # "单列扫描"
                            n208 = local read "开关控制器"() -> (w437:refnum<visa-resource-name>)
                            n209 = local read "频率步进次数"() -> (w436:dbl)
                            n210 = Write to Text File(file (use dialog)=w434, text=w432) -> (refnum out=w433:refnum<file>)  [unwired: 2 in, 2 out]
                            n211 = for {
                              N: w436 -> [_]
                              tunnel: w437 -> [w447]
                              tunnel: w433 -> [w444]
                              tunnel: [w442] -> w440
                              tunnel: [w441] -> w435
                              i -> [w446]
                              n212 = flat-sequence {
                                tunnel: w447 -> [w454]
                                tunnel: w446 -> [w450]
                                tunnel: [w452] -> w445
                                tunnel: w444 -> [w448]
                                tunnel: [w448] -> w443
                                tunnel: w445 -> [w467]
                                tunnel: w443 -> [w475]
                                tunnel: [w464] -> w442
                                tunnel: [w463] -> w441
                                frame #0 {
                                # "初始化"
                                n213 = local read "频率间隔"() -> (w451:dbl)
                                n214 = Multiply(x=w450, y=w451) -> (x*y=w462:dbl)
                                n215 = Add(x=w462, y=24) -> (x+y=w449:dbl)
                                n216 = call "freqToVolt.vi"("频率"=w449) -> ("电压"=w456:dbl)
                                n217 = Number To Decimal String(number=w456) -> (decimal integer string=w459:string)  [unwired: 1 in]
                                n218 = Concatenate Strings("v", w459, "\r\n") -> (w457:string)
                                n219 = local write "当前频率"(w449) -> ()
                                n220 = VISA Write(VISA resource name=w454, write buffer=w457) -> (VISA resource name out=w453:refnum<visa-resource-name>)  [unwired: 1 in, 2 out]
                                n221 = VISA Read(VISA resource name=w453, byte count=6) -> (VISA resource name out=w452:refnum<visa-resource-name>)  [unwired: 1 in, 3 out]
                                }
                                frame #1 {
                                w476 = "\r\n"
                                # "扫描"
                                n222 = dll-call lib="C:/Users/BlueMess/Desktop/Work2020/MMW Controller/mmw_controller/PCI8552B_32.dll" fn="PCI8552B_CreateDevice" label="CreateDevice"("DeviceLgcID"=0) -> ("返回类型"=w473:i32)  [unwired: 4 in, 2 out]
                                n223 = call "artInitParm.vi"() -> ("待读取长度"=w469:dbl, "量程选择"=w470:dbl, "初始化参数"=w474:dbl[])
                                n224 = dll-call lib="C:/Users/BlueMess/Desktop/Work2020/MMW Controller/mmw_controller/PCI8552B_32.DLL" fn="PCI8552B_InitDeviceAD" label="InitDeviceAD"("hDevice"=w473, "pADPara"=w474) -> ("hDevice"=w471:i32)  [unwired: 5 in, 2 out]
                                n225 = for {
                                N: 31 -> [_]
                                tunnel: w467 -> [w491]
                                tunnel: w471 -> [w487]
                                tunnel: w469 -> [w485]
                                tunnel: w470 -> [w483]
                                tunnel: [w482] -> w464
                                tunnel: [w481] -> w465 mode=indexing
                                tunnel: [w480] -> w466 mode=indexing
                                i -> [w490]
                                n226 = flat-sequence {
                                tunnel: w491 -> [w504]
                                tunnel: w490 -> [w492]
                                tunnel: [w499] -> w489
                                tunnel: [w496] -> w488
                                tunnel: w487 -> [w496]
                                tunnel: [w495] -> w486
                                tunnel: w485 -> [w495]
                                tunnel: [w494] -> w484
                                tunnel: w483 -> [w494]
                                tunnel: w489 -> [_]
                                tunnel: w488 -> [w511]
                                tunnel: w486 -> [w512]
                                tunnel: w484 -> [w505]
                                tunnel: [w510] -> w482
                                tunnel: [w509] -> w481
                                tunnel: [w508] -> w480
                                frame #0 {
                                n227 = Number To Decimal String(number=w492) -> (decimal integer string=w503:string)  [unwired: 1 in]
                                n228 = Increment(x=w492) -> (x+1=w493:i32)
                                n229 = Concatenate Strings("k", w503, "\r\n") -> (w500:string)
                                n230 = local write "当前开关"(w493) -> ()
                                n231 = VISA Write(VISA resource name=w504, write buffer=w500) -> (VISA resource name out=w498:refnum<visa-resource-name>)  [unwired: 1 in, 2 out]
                                n232 = VISA Read(VISA resource name=w498, byte count=6) -> (VISA resource name out=w499:refnum<visa-resource-name>)  [unwired: 1 in, 3 out]
                                }
                                frame #1 {
                                n233 = local write "待读取数据长度"(w505) -> ()
                                n234 = stacked-sequence {
                                tunnel: w511 -> [w514 w545]
                                tunnel: [_ w549] -> w510
                                tunnel: w512 -> [_ w544]
                                tunnel: [_ w543] -> w507
                                tunnel: [_ w542] -> w506
                                frame #0 {
                                n235 = dll-call lib="C:/Users/BlueMess/Desktop/Work2020/MMW Controller/mmw_controller/PCI8552B_32.DLL" fn="PCI8552B_StartDeviceAD" label="StartDeviceAD"("hDevice"=w514) -> ("hDevice"=w513:i32)  [unwired: 4 in, 2 out]
                                n236 = Initialize Array(0, 5) -> (w518:i32[])
                                n237 = while {
                                tunnel: w513 -> [w522]
                                tunnel: w518 -> [w527]
                                tunnel: [w520] -> w515
                                stop <- w519 stop-if-true
                                n238 = dll-call lib="C:/Users/BlueMess/Desktop/Work2020/MMW Controller/mmw_controller/PCI8552B_32.DLL" fn="PCI8552B_SetDeviceTrigAD" label="SetDeviceTrigAD"("hDevice"=w522) -> ("hDevice"=w521:i32)  [unwired: 4 in, 2 out]
                                n239 = dll-call lib="C:/Users/BlueMess/Desktop/Work2020/MMW Controller/mmw_controller/PCI8552B_32.DLL" fn="PCI8552B_GetDevStatusAD" label="GetDevStatusAD"("hDevice"=w521, "ADStatus"=w527) -> ("hDevice"=w520:i32, "ADStatus"=w523:i32[])  [unwired: 4 in, 2 out]
                                n240 = Index Array(array=w523, index=2) -> (element=w525:i32)
                                n241 = Equal?(x=1, y=w525) -> (x = y?=w519:bool)
                                }
                                n242 = dll-call lib="C:/Users/BlueMess/Desktop/Work2020/MMW Controller/mmw_controller/PCI8552B_32.DLL" fn="PCI8552B_StopDeviceAD" label="StopDeviceAD"("hDevice"=w515) -> ()  [unwired: 5 in, 2 out]
                                }
                                frame #1 {
                                n243 = local read "待读取数据长度"() -> (w539:i32)
                                n244 = Initialize Array(u16 0 ("y"), 2048 ("y")) -> (w546:u16[])
                                n245 = local read "待读取数据长度"() -> (w538:i32)
                                n246 = Greater Or Equal?(x=w539, y=2048 ("millisecond multiple")) -> (x >= y?=w540:bool)
                                n247 = case shown="真" w540 {
                                tunnel: [w568 2048 ("millisecond multiple")] -> w536
                                tunnel: w539 -> [w568 _]
                                frame False {
                                }
                                frame True {
                                }
                                }
                                n248 = dll-call lib="C:/Users/BlueMess/Desktop/Work2020/MMW Controller/mmw_controller/PCI8552B_32.DLL" fn="PCI8552B_ReadDeviceAD" label="ReadDeviceAD"("hDevice"=w545, "pADBuffer"=w546, "nReadSizeWords"=w536, "nRetSizeWords"=0) -> ("hDevice"=w549:i32, "pADBuffer"=w531:u16[], "nReadSizeWords"=w528:u32)  [unwired: 5 in, 2 out]
                                n249 = Subtract(x=w538, y=w528) -> (x-y=w537:u32)
                                n250 = local write "待读取数据长度"(w537) -> ()
                                n251 = Array Subset(array=w531, index=0 ("索引"), length=w528) -> (w530:u16[])
                                n252 = And(x=w530, y=u16 4095) -> (x .and. y?=w534:u16[])
                                n253 = case shown="1" w544 {
                                tunnel: w534 -> [w557 w562]
                                tunnel: [w550 w561] -> w533
                                frame 0, Default {
                                n254 = To Double Precision Float(number=2000 ("x")) -> (double precision float=w553:dbl)
                                n255 = To Double Precision Float(number=4096) -> (double precision float=w552:dbl)
                                n256 = Divide(x=w553, y=w552) -> (x/y=w558:dbl)
                                n257 = Multiply(x=w558, y=w557) -> (x*y=w556:dbl[])
                                n258 = Subtract(x=w556, y=1000.0) -> (x-y=w550:dbl[])
                                }
                                frame 1 {
                                n259 = To Double Precision Float(number=10000 ("x")) -> (double precision float=w560:dbl)
                                n260 = To Double Precision Float(number=4096) -> (double precision float=w564:dbl)
                                n261 = Divide(x=w560, y=w564) -> (x/y=w567:dbl)
                                n262 = Multiply(x=w567, y=w562) -> (x*y=w566:dbl[])
                                n263 = Subtract(x=w566, y=5000.0) -> (x-y=w561:dbl[])
                                }
                                }
                                n264 = Decimate 1D Array(w533) -> (w543:dbl[], w542:dbl[])
                                }
                                }
                                n265 = call "dataProcessing.vi"("中频信号"=w506, "参考信号"=w507) -> ("mean_Q"=w508:dbl, "mean_I"=w509:dbl)
                                n266 = local write "ch1"(w506) -> ()
                                n267 = local write "ch0"(w507) -> ()
                                }
                                }
                                }
                                n268 = call "numArray2String.vi"("输入数组"=w465) -> ("输出字符串"=w477:string)
                                n269 = call "numArray2String.vi"("输入数组"=w466) -> ("输出字符串"=w478:string)
                                n270 = Concatenate Strings(w477, w476, w478, w476) -> (w479:string)
                                n271 = Write to Text File(file (use dialog)=w475, text=w479) -> (refnum out=w463:refnum<file>)  [unwired: 2 in, 2 out]
                                }
                              }
                            }
                            n272 = dll-call lib="C:/Users/BlueMess/Desktop/Work2020/MMW Controller/mmw_controller/PCI8552B_32.DLL" fn="PCI8552B_StopDeviceAD" label="StopDeviceAD"("hDevice"=w440) -> ("hDevice"=w439:i32)  [unwired: 4 in, 2 out]
                            n273 = dll-call lib="C:/Users/BlueMess/Desktop/Work2020/MMW Controller/mmw_controller/PCI8552B_32.DLL" fn="PCI8552B_ReleaseDeviceAD" label="ReleaseDeviceAD"("hDevice"=w439) -> ("hDevice"=w438:i32)  [unwired: 4 in, 2 out]
                            n274 = dll-call lib="C:/Users/BlueMess/Desktop/Work2020/MMW Controller/mmw_controller/PCI8552B_32.DLL" fn="PCI8552B_ReleaseDevice" label="ReleaseDevice"("hDevice"=w438) -> ()  [unwired: 5 in, 2 out]
                          }
                        }
                      }
                      frame 2 {
                        # "单点模式"
                        n275 = call "singlePointMode.vi"() -> ("ch1"=w571:dbl[], "ch0"=w570:dbl[])
                        n276 = local write "ch1"(w571) -> ()
                        n277 = local write "ch0"(w570) -> ()
                      }
                      frame 3 {
                        # "单列模式"
                        n278 = local read "频率步进次数"() -> (w578:dbl)
                        n279 = local read "开关控制器"() -> (w577:refnum<visa-resource-name>)
                        n280 = for {
                          N: w578 -> [_]
                          tunnel: w577 -> [w585]
                          tunnel: w576 -> [w582]
                          tunnel: [w580] -> w573
                          tunnel: [w579] -> w572
                          i -> [w584]
                          n281 = flat-sequence {
                            tunnel: w585 -> [w597]
                            tunnel: w584 -> [w593]
                            tunnel: [w595] -> w583
                            tunnel: w582 -> [w591]
                            tunnel: [w590] -> w581
                            tunnel: w583 -> [w610]
                            tunnel: w581 -> [w618]
                            tunnel: [w607] -> w580
                            tunnel: [w606] -> w579
                            frame #0 {
                              # "初始化"
                              n282 = local read "频率间隔"() -> (w594:dbl)
                              n283 = local read "步进间隔"() -> (w587:dbl)
                              n284 = local read "频率间隔"() -> (w586:dbl)
                              n285 = local read "物体距离"() -> (w588:dbl)
                              n286 = Multiply(x=w593, y=w594) -> (x*y=w605:dbl)
                              n287 = Add(x=w605, y=24) -> (x+y=w592:dbl)
                              n288 = call "fileHead.vi"("df"=w586, "dx"=w587, "distance"=w588) -> ("输出"=w589:string)  [unwired: 6 in]
                              n289 = call "freqToVolt.vi"("频率"=w592) -> ("电压"=w599:dbl)
                              n290 = Write to Text File(file (use dialog)=w591, text=w589) -> (refnum out=w590:refnum<file>)  [unwired: 2 in, 2 out]
                              n291 = Number To Decimal String(number=w599) -> (decimal integer string=w602:string)  [unwired: 1 in]
                              n292 = Concatenate Strings("v", w602, "\r\n") -> (w600:string)
                              n293 = local write "当前频率"(w592) -> ()
                              n294 = VISA Write(VISA resource name=w597, write buffer=w600) -> (VISA resource name out=w596:refnum<visa-resource-name>)  [unwired: 1 in, 2 out]
                              n295 = VISA Read(VISA resource name=w596, byte count=6) -> (VISA resource name out=w595:refnum<visa-resource-name>)  [unwired: 1 in, 3 out]
                            }
                            frame #1 {
                              w619 = "\r\n"
                              # "扫描"
                              n296 = dll-call lib="C:/Users/BlueMess/Desktop/Work2020/MMW Controller/mmw_controller/PCI8552B_32.dll" fn="PCI8552B_CreateDevice" label="CreateDevice"("DeviceLgcID"=0) -> ("返回类型"=w616:i32)  [unwired: 4 in, 2 out]
                              n297 = call "artInitParm.vi"() -> ("待读取长度"=w612:dbl, "量程选择"=w613:dbl, "初始化参数"=w617:dbl[])
                              n298 = dll-call lib="C:/Users/BlueMess/Desktop/Work2020/MMW Controller/mmw_controller/PCI8552B_32.DLL" fn="PCI8552B_InitDeviceAD" label="InitDeviceAD"("hDevice"=w616, "pADPara"=w617) -> ("hDevice"=w614:i32)  [unwired: 5 in, 2 out]
                              n299 = for {
                                N: 31 -> [_]
                                tunnel: w610 -> [w634]
                                tunnel: w614 -> [w630]
                                tunnel: w612 -> [w628]
                                tunnel: w613 -> [w626]
                                tunnel: [w625] -> w607
                                tunnel: [w624] -> w608 mode=indexing
                                tunnel: [w623] -> w609 mode=indexing
                                i -> [w633]
                                n300 = flat-sequence {
                                tunnel: w634 -> [w647]
                                tunnel: w633 -> [w635]
                                tunnel: [w642] -> w632
                                tunnel: [w639] -> w631
                                tunnel: w630 -> [w639]
                                tunnel: [w638] -> w629
                                tunnel: w628 -> [w638]
                                tunnel: [w637] -> w627
                                tunnel: w626 -> [w637]
                                tunnel: w632 -> [_]
                                tunnel: w631 -> [w654]
                                tunnel: w629 -> [w655]
                                tunnel: w627 -> [w653]
                                tunnel: [w652] -> w625
                                tunnel: [w651] -> w624
                                tunnel: [w650] -> w623
                                frame #0 {
                                n301 = Number To Decimal String(number=w635) -> (decimal integer string=w646:string)  [unwired: 1 in]
                                n302 = Concatenate Strings("k", w646, "\r\n") -> (w643:string)
                                n303 = Increment(x=w635) -> (x+1=w636:i32)
                                n304 = VISA Write(VISA resource name=w647, write buffer=w643) -> (VISA resource name out=w641:refnum<visa-resource-name>)  [unwired: 1 in, 2 out]
                                n305 = local write "当前开关"(w636) -> ()
                                n306 = VISA Read(VISA resource name=w641, byte count=6) -> (VISA resource name out=w642:refnum<visa-resource-name>)  [unwired: 1 in, 3 out]
                                }
                                frame #1 {
                                n307 = stacked-sequence {
                                tunnel: w654 -> [w657 w688]
                                tunnel: [_ w692] -> w652
                                tunnel: w655 -> [_ w687]
                                tunnel: [_ w686] -> w649
                                tunnel: [_ w685] -> w648
                                frame #0 {
                                n308 = dll-call lib="C:/Users/BlueMess/Desktop/Work2020/MMW Controller/mmw_controller/PCI8552B_32.DLL" fn="PCI8552B_StartDeviceAD" label="StartDeviceAD"("hDevice"=w657) -> ("hDevice"=w656:i32)  [unwired: 4 in, 2 out]
                                n309 = Initialize Array(0, 5) -> (w661:i32[])
                                n310 = while {
                                tunnel: w656 -> [w665]
                                tunnel: w661 -> [w670]
                                tunnel: [w663] -> w658
                                stop <- w662 stop-if-true
                                n311 = dll-call lib="C:/Users/BlueMess/Desktop/Work2020/MMW Controller/mmw_controller/PCI8552B_32.DLL" fn="PCI8552B_SetDeviceTrigAD" label="SetDeviceTrigAD"("hDevice"=w665) -> ("hDevice"=w664:i32)  [unwired: 4 in, 2 out]
                                n312 = dll-call lib="C:/Users/BlueMess/Desktop/Work2020/MMW Controller/mmw_controller/PCI8552B_32.DLL" fn="PCI8552B_GetDevStatusAD" label="GetDevStatusAD"("hDevice"=w664, "ADStatus"=w670) -> ("hDevice"=w663:i32, "ADStatus"=w666:i32[])  [unwired: 4 in, 2 out]
                                n313 = Index Array(array=w666, index=2) -> (element=w668:i32)
                                n314 = Equal?(x=1, y=w668) -> (x = y?=w662:bool)
                                }
                                n315 = dll-call lib="C:/Users/BlueMess/Desktop/Work2020/MMW Controller/mmw_controller/PCI8552B_32.DLL" fn="PCI8552B_StopDeviceAD" label="StopDeviceAD"("hDevice"=w658) -> ()  [unwired: 5 in, 2 out]
                                }
                                frame #1 {
                                n316 = local read "待读取数据长度"() -> (w682:i32)
                                n317 = local read "待读取数据长度"() -> (w681:i32)
                                n318 = Initialize Array(u16 0 ("y"), 2048 ("y")) -> (w689:u16[])
                                n319 = Greater Or Equal?(x=w682, y=2048 ("millisecond multiple")) -> (x >= y?=w683:bool)
                                n320 = case shown="真" w683 {
                                tunnel: [w711 2048 ("millisecond multiple")] -> w679
                                tunnel: w682 -> [w711 _]
                                frame False {
                                }
                                frame True {
                                }
                                }
                                n321 = dll-call lib="C:/Users/BlueMess/Desktop/Work2020/MMW Controller/mmw_controller/PCI8552B_32.DLL" fn="PCI8552B_ReadDeviceAD" label="ReadDeviceAD"("hDevice"=w688, "pADBuffer"=w689, "nReadSizeWords"=w679, "nRetSizeWords"=0) -> ("hDevice"=w692:i32, "pADBuffer"=w674:u16[], "nReadSizeWords"=w671:u32)  [unwired: 5 in, 2 out]
                                n322 = Subtract(x=w681, y=w671) -> (x-y=w680:u32)
                                n323 = Array Subset(array=w674, index=0 ("索引"), length=w671) -> (w673:u16[])
                                n324 = local write "待读取数据长度"(w680) -> ()
                                n325 = And(x=w673, y=u16 4095) -> (x .and. y?=w677:u16[])
                                n326 = case shown="1" w687 {
                                tunnel: w677 -> [w700 w705]
                                tunnel: [w693 w704] -> w676
                                frame 0, Default {
                                n327 = To Double Precision Float(number=2000 ("x")) -> (double precision float=w696:dbl)
                                n328 = To Double Precision Float(number=4096) -> (double precision float=w695:dbl)
                                n329 = Divide(x=w696, y=w695) -> (x/y=w701:dbl)
                                n330 = Multiply(x=w701, y=w700) -> (x*y=w699:dbl[])
                                n331 = Subtract(x=w699, y=1000.0) -> (x-y=w693:dbl[])
                                }
                                frame 1 {
                                n332 = To Double Precision Float(number=10000 ("x")) -> (double precision float=w703:dbl)
                                n333 = To Double Precision Float(number=4096) -> (double precision float=w707:dbl)
                                n334 = Divide(x=w703, y=w707) -> (x/y=w710:dbl)
                                n335 = Multiply(x=w710, y=w705) -> (x*y=w709:dbl[])
                                n336 = Subtract(x=w709, y=5000.0) -> (x-y=w704:dbl[])
                                }
                                }
                                n337 = Decimate 1D Array(w676) -> (w686:dbl[], w685:dbl[])
                                }
                                }
                                n338 = call "dataProcessing.vi"("中频信号"=w648, "参考信号"=w649) -> ("mean_Q"=w650:dbl, "mean_I"=w651:dbl)
                                n339 = local write "ch0"(w649) -> ()
                                n340 = local write "ch1"(w648) -> ()
                                "待读取数据长度" <- w653
                                }
                                }
                              }
                              n341 = call "numArray2String.vi"("输入数组"=w609) -> ("输出字符串"=w621:string)
                              n342 = call "numArray2String.vi"("输入数组"=w608) -> ("输出字符串"=w620:string)
                              n343 = Concatenate Strings(w620, w619, w621, w619) -> (w622:string)
                              n344 = Write to Text File(file (use dialog)=w618, text=w622) -> (refnum out=w606:refnum<file>)  [unwired: 2 in, 2 out]
                            }
                          }
                        }
                        n345 = dll-call lib="C:/Users/BlueMess/Desktop/Work2020/MMW Controller/mmw_controller/PCI8552B_32.DLL" fn="PCI8552B_StopDeviceAD" label="StopDeviceAD"("hDevice"=w573) -> ("hDevice"=w574:i32)  [unwired: 4 in, 2 out]
                        n346 = dll-call lib="C:/Users/BlueMess/Desktop/Work2020/MMW Controller/mmw_controller/PCI8552B_32.DLL" fn="PCI8552B_ReleaseDeviceAD" label="ReleaseDeviceAD"("hDevice"=w574) -> ("hDevice"=w575:i32)  [unwired: 4 in, 2 out]
                        n347 = dll-call lib="C:/Users/BlueMess/Desktop/Work2020/MMW Controller/mmw_controller/PCI8552B_32.DLL" fn="PCI8552B_ReleaseDevice" label="ReleaseDevice"("hDevice"=w575) -> ()  [unwired: 5 in, 2 out]
                      }
                      frame 4 {
                        w714 = 0
                        w737 = "\r\n"
                        # "单频多角度模式"
                        n348 = local read "物体距离"() -> (w716:dbl)
                        n349 = local read "当前位置"() -> (w715:dbl)
                        n350 = local read "当前频率"() -> (w713:dbl)
                        n351 = local read "开关控制器"() -> (w735:refnum<visa-resource-name>)
                        n352 = dll-call lib="C:/Users/BlueMess/Desktop/Work2020/MMW Controller/mmw_controller/PCI8552B_32.dll" fn="PCI8552B_CreateDevice" label="CreateDevice"("DeviceLgcID"=0) -> ("返回类型"=w733:i32)  [unwired: 4 in, 2 out]
                        n353 = call "artInitParm.vi"() -> ("待读取长度"=w729:dbl, "量程选择"=w730:dbl, "初始化参数"=w734:dbl[])
                        n354 = call "fileHead.vi"("df"=w714, "f_min"=w713, "f_max"=w713, "x_max"=w715, "dx"=w714, "x_min"=w715, "distance"=w716) -> ("输出"=w717:string)  [unwired: 2 in]
                        n355 = Write to Text File(file (use dialog)=w719, text=w717) -> (refnum out=w718:refnum<file>)  [unwired: 2 in, 2 out]
                        n356 = dll-call lib="C:/Users/BlueMess/Desktop/Work2020/MMW Controller/mmw_controller/PCI8552B_32.DLL" fn="PCI8552B_InitDeviceAD" label="InitDeviceAD"("hDevice"=w733, "pADPara"=w734) -> ("hDevice"=w731:i32)  [unwired: 5 in, 2 out]
                        n357 = for {
                          N: 31 -> [_]
                          tunnel: w735 -> [w750]
                          tunnel: [w749] -> _
                          tunnel: w731 -> [w745]
                          tunnel: w730 -> [w743]
                          tunnel: w729 -> [w741]
                          tunnel: [w740] -> w724
                          tunnel: [w739] -> w728 mode=indexing
                          tunnel: [w738] -> w727 mode=indexing
                          i -> [w748]
                          n358 = flat-sequence {
                            tunnel: w750 -> [w763]
                            tunnel: w748 -> [w752]
                            tunnel: [w758] -> w747
                            tunnel: [w755] -> w746
                            tunnel: w745 -> [w755]
                            tunnel: [w754] -> w744
                            tunnel: w743 -> [w754]
                            tunnel: [w753] -> w742
                            tunnel: w741 -> [w753]
                            tunnel: [w772] -> w749
                            tunnel: w747 -> [w772]
                            tunnel: w746 -> [w770]
                            tunnel: w744 -> [w771]
                            tunnel: w742 -> [w764]
                            tunnel: [w769] -> w740
                            tunnel: [w768] -> w739
                            tunnel: [w767] -> w738
                            frame #0 {
                              n359 = Number To Decimal String(number=w752) -> (decimal integer string=w762:string)  [unwired: 1 in]
                              n360 = Concatenate Strings("k", w762, "\r\n") -> (w759:string)
                              n361 = Increment(x=w752) -> (x+1=w751:i32)
                              n362 = VISA Write(VISA resource name=w763, write buffer=w759) -> (VISA resource name out=w757:refnum<visa-resource-name>)  [unwired: 1 in, 2 out]
                              n363 = local write "当前开关"(w751) -> ()
                              n364 = VISA Read(VISA resource name=w757, byte count=6) -> (VISA resource name out=w758:refnum<visa-resource-name>)  [unwired: 1 in, 3 out]
                            }
                            frame #1 {
                              n365 = local write "待读取数据长度"(w764) -> ()
                              n366 = stacked-sequence {
                                tunnel: w770 -> [w774 w805]
                                tunnel: [_ w809] -> w769
                                tunnel: w771 -> [_ w804]
                                tunnel: [_ w803] -> w766
                                tunnel: [_ w802] -> w765
                                frame #0 {
                                n367 = dll-call lib="C:/Users/BlueMess/Desktop/Work2020/MMW Controller/mmw_controller/PCI8552B_32.DLL" fn="PCI8552B_StartDeviceAD" label="StartDeviceAD"("hDevice"=w774) -> ("hDevice"=w773:i32)  [unwired: 4 in, 2 out]
                                n368 = Initialize Array(0, 5) -> (w778:i32[])
                                n369 = while {
                                tunnel: w773 -> [w782]
                                tunnel: w778 -> [w787]
                                tunnel: [w780] -> w775
                                stop <- w779 stop-if-true
                                n370 = dll-call lib="C:/Users/BlueMess/Desktop/Work2020/MMW Controller/mmw_controller/PCI8552B_32.DLL" fn="PCI8552B_SetDeviceTrigAD" label="SetDeviceTrigAD"("hDevice"=w782) -> ("hDevice"=w781:i32)  [unwired: 4 in, 2 out]
                                n371 = dll-call lib="C:/Users/BlueMess/Desktop/Work2020/MMW Controller/mmw_controller/PCI8552B_32.DLL" fn="PCI8552B_GetDevStatusAD" label="GetDevStatusAD"("hDevice"=w781, "ADStatus"=w787) -> ("hDevice"=w780:i32, "ADStatus"=w783:i32[])  [unwired: 4 in, 2 out]
                                n372 = Index Array(array=w783, index=2) -> (element=w785:i32)
                                n373 = Equal?(x=1, y=w785) -> (x = y?=w779:bool)
                                }
                                n374 = dll-call lib="C:/Users/BlueMess/Desktop/Work2020/MMW Controller/mmw_controller/PCI8552B_32.DLL" fn="PCI8552B_StopDeviceAD" label="StopDeviceAD"("hDevice"=w775) -> ()  [unwired: 5 in, 2 out]
                                }
                                frame #1 {
                                n375 = local read "待读取数据长度"() -> (w799:i32)
                                n376 = Initialize Array(u16 0 ("y"), 2048 ("y")) -> (w806:u16[])
                                n377 = Greater Or Equal?(x=w799, y=2048 ("millisecond multiple")) -> (x >= y?=w800:bool)
                                n378 = case shown="假" w800 {
                                tunnel: [w828 2048 ("millisecond multiple")] -> w796
                                tunnel: w799 -> [w828 _]
                                frame False {
                                }
                                frame True {
                                }
                                }
                                n379 = dll-call lib="C:/Users/BlueMess/Desktop/Work2020/MMW Controller/mmw_controller/PCI8552B_32.DLL" fn="PCI8552B_ReadDeviceAD" label="ReadDeviceAD"("hDevice"=w805, "pADBuffer"=w806, "nReadSizeWords"=w796, "nRetSizeWords"=0) -> ("hDevice"=w809:i32, "pADBuffer"=w791:u16[], "nReadSizeWords"=w788:u32)  [unwired: 5 in, 2 out]
                                n380 = Array Subset(array=w791, index=0 ("索引"), length=w788) -> (w790:u16[])
                                n381 = local read "待读取数据长度"() -> (w798:i32)
                                n382 = And(x=w790, y=u16 4095) -> (x .and. y?=w794:u16[])
                                n383 = Subtract(x=w798, y=w788) -> (x-y=w797:u32)
                                n384 = case shown="1" w804 {
                                tunnel: w794 -> [w817 w822]
                                tunnel: [w810 w821] -> w793
                                frame 0, Default {
                                n385 = To Double Precision Float(number=2000 ("x")) -> (double precision float=w813:dbl)
                                n386 = To Double Precision Float(number=4096) -> (double precision float=w812:dbl)
                                n387 = Divide(x=w813, y=w812) -> (x/y=w818:dbl)
                                n388 = Multiply(x=w818, y=w817) -> (x*y=w816:dbl[])
                                n389 = Subtract(x=w816, y=1000.0) -> (x-y=w810:dbl[])
                                }
                                frame 1 {
                                n390 = To Double Precision Float(number=10000 ("x")) -> (double precision float=w820:dbl)
                                n391 = To Double Precision Float(number=4096) -> (double precision float=w824:dbl)
                                n392 = Divide(x=w820, y=w824) -> (x/y=w827:dbl)
                                n393 = Multiply(x=w827, y=w822) -> (x*y=w826:dbl[])
                                n394 = Subtract(x=w826, y=5000.0) -> (x-y=w821:dbl[])
                                }
                                }
                                n395 = local write "待读取数据长度"(w797) -> ()
                                n396 = Decimate 1D Array(w793) -> (w803:dbl[], w802:dbl[])
                                }
                              }
                              n397 = local write "ch1"(w765) -> ()
                              n398 = call "dataProcessing.vi"("中频信号"=w765, "参考信号"=w766) -> ("mean_Q"=w767:dbl, "mean_I"=w768:dbl)
                              n399 = local write "ch0"(w766) -> ()
                            }
                          }
                        }
                        n400 = dll-call lib="C:/Users/BlueMess/Desktop/Work2020/MMW Controller/mmw_controller/PCI8552B_32.DLL" fn="PCI8552B_StopDeviceAD" label="StopDeviceAD"("hDevice"=w724) -> ("hDevice"=w726:i32)  [unwired: 4 in, 2 out]
                        n401 = call "numArray2String.vi"("输入数组"=w728) -> ("输出字符串"=w721:string)
                        n402 = call "numArray2String.vi"("输入数组"=w727) -> ("输出字符串"=w720:string)
                        n403 = dll-call lib="C:/Users/BlueMess/Desktop/Work2020/MMW Controller/mmw_controller/PCI8552B_32.DLL" fn="PCI8552B_ReleaseDeviceAD" label="ReleaseDeviceAD"("hDevice"=w726) -> ("hDevice"=w725:i32)  [unwired: 4 in, 2 out]
                        n404 = dll-call lib="C:/Users/BlueMess/Desktop/Work2020/MMW Controller/mmw_controller/PCI8552B_32.DLL" fn="PCI8552B_ReleaseDevice" label="ReleaseDevice"("hDevice"=w725) -> ()  [unwired: 5 in, 2 out]
                        n405 = Concatenate Strings(w721, w737, w720, w737) -> (w736:string)
                        n406 = Write to Text File(file (use dialog)=w718, text=w736) -> (refnum out=w723:refnum<file>)  [unwired: 2 in, 2 out]
                      }
                    }
                  }
                }
              }
            }
          }
        }
        n407 = Or(x=w45, y="停止") -> (x .or. y?=w43:bool)
      }
    }
  }
